vi "Kafka_ConsumerSeek.vi"(8 "error in (no error)":errorcluster, 10 "offset":i64, 11 "Producer Handle":string="localhost:9092") -> (0 "error out":errorcluster, 3 "Producer Handle":string)   [LabVIEW 2019, in "LVKafka.lvlib"]
uses:
  LVKafka.lvlib
  KafkaLVLib.dll
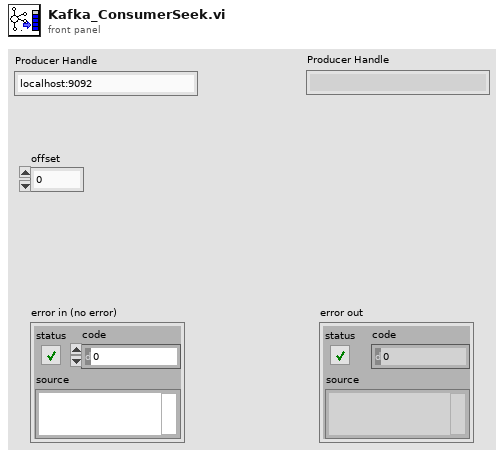
[diagram p1: front panel]
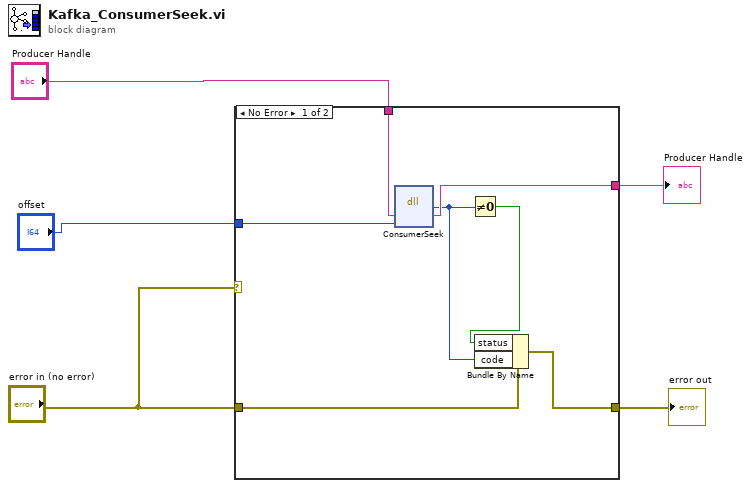
[diagram p0: block diagram]
diagram:
  n1 = case shown="No Error" "error in (no error)" {
    tunnel: "Producer Handle" -> [w12 w14]
    tunnel: [w11 w13] -> w4
    tunnel: [w10 w14] -> w3
    tunnel: "error in (no error)" -> [w7 w13]
    tunnel: "offset" -> [w6 _]
    frame No Error {
      n2 = dll-call lib="KafkaLVLib.*" fn="ConsumerSeek"("producerhandle"=w12, "offset"=w6) -> ("error"=w8:i32, "producerhandle"=w10:string)  [unwired: 4 in, 2 out]
      n3 = Not Equal To 0?(x=w8) -> (x != 0?=w9:bool)
      n4 = Bundle By Name(cluster=w7, "status"=w9, "code"=w8) -> (w11:errorcluster)
    }
    frame Error {
    }
  }
  "error out" <- w4
  "Producer Handle" <- w3
